vi "Save.vi"(8 "error in (no error)":errorcluster, 10 "File Path":path, 11 "Excel in":refnum<class "Excel.lvclass">) -> (0 "error out":errorcluster, 2 "Cancelled?":bool, 3 "Excel out":refnum<class "Excel.lvclass">)   [LabVIEW 2016, in "Excel.lvclass"]
doc: "Saves the Excel workbook referenced by the Excel input class.\n\nIf a file path is provided the workbook will be saved to that path overwriting existing files.\nIf a file path is not provided but the workbook has previously been saved the workbook will be saved to it's existing location.\nIf neither of the above are true the user will be prompted for a file path and if a file already exists at that path will be prompted again to ensure they want to overwrite the existing file.\n\nCancelled is returned as true if the file is not saved for any reason including an input error."
uses:
  Excel.lvclass
  Excel.lvclass/Excel.ctl
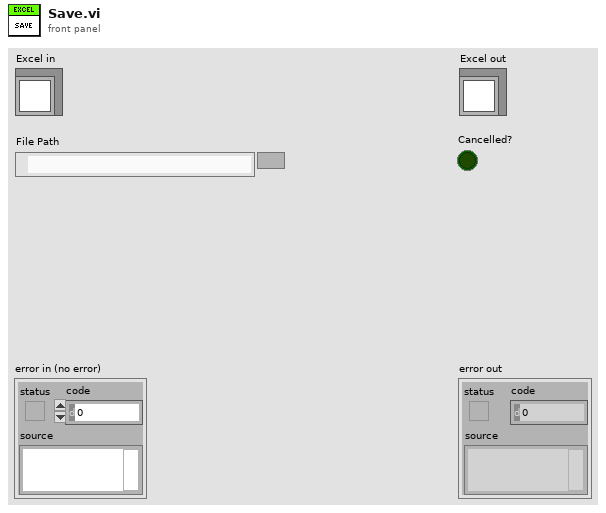
[diagram p1: front panel]
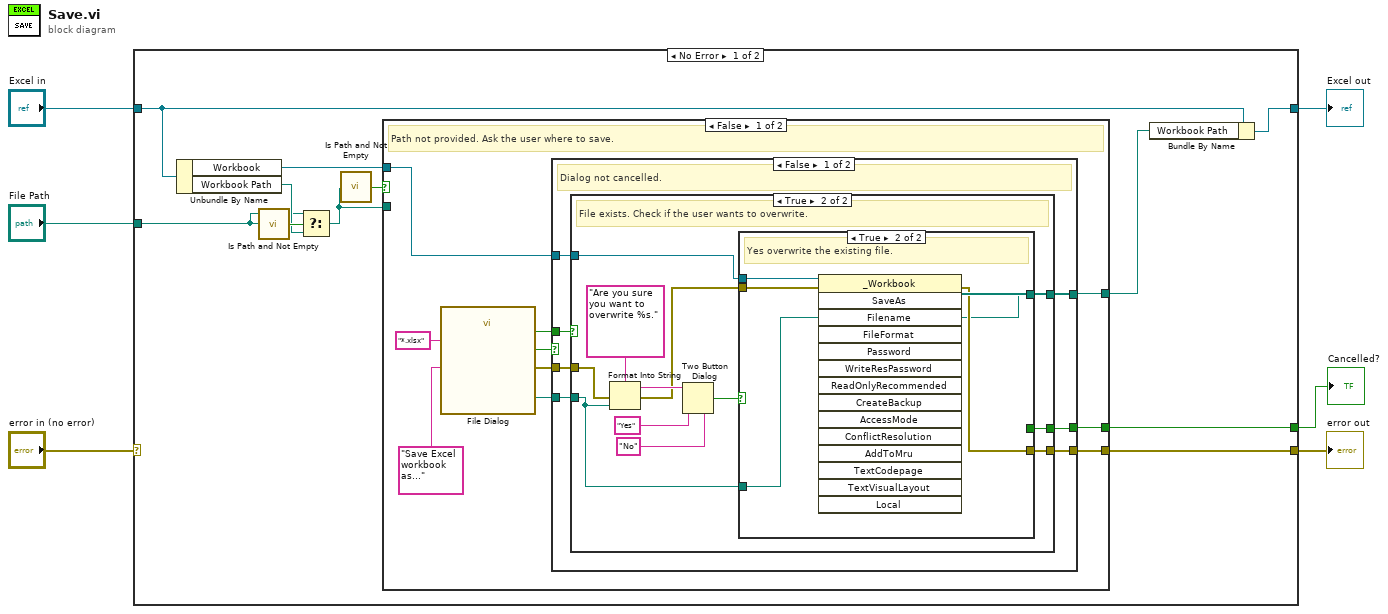
[diagram p0: block diagram]
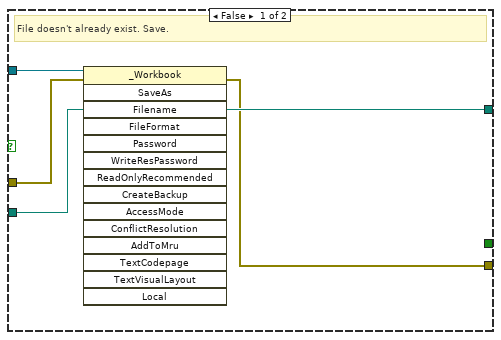
[diagram p2: hidden frame]
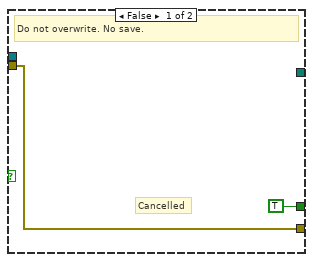
[diagram p3: hidden frame]
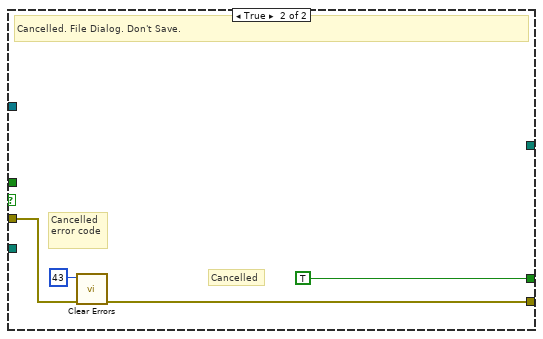
[diagram p4: hidden frame]
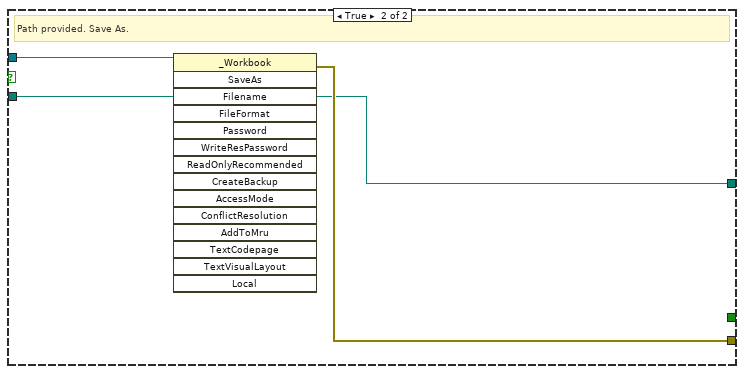
[diagram p5: hidden frame]
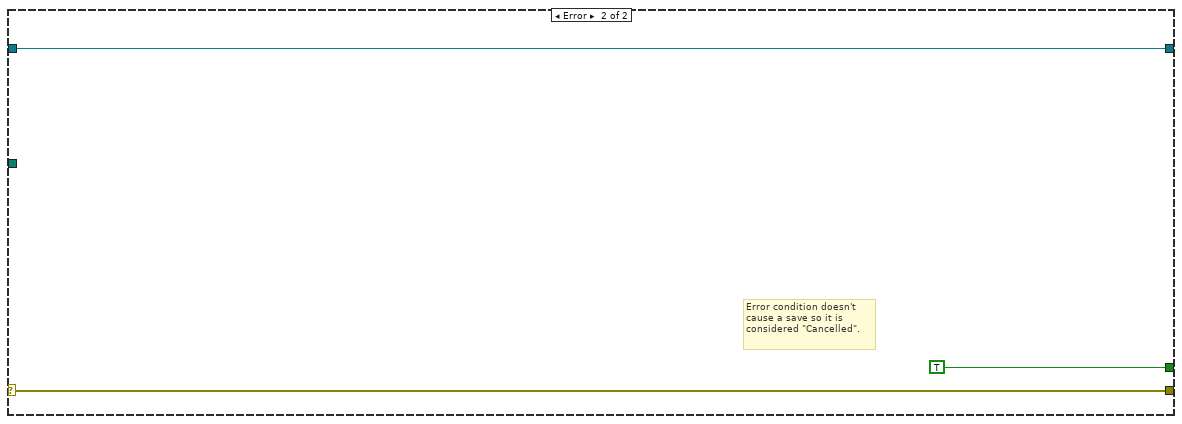
[diagram p6: hidden frame]
diagram:
  n1 = case shown="No Error" "error in (no error)" {
    selector: "error in (no error)" -> [_ w66]
    tunnel: [w13 w66] -> w5
    tunnel: [w16 w65] -> w3
    tunnel: "Excel in" -> [w17 w65]
    tunnel: "File Path" -> [w10 _]
    tunnel: [w7 TRUE] -> w1
    frame No Error {
      n2 = Unbundle By Name(w17) -> ("Workbook"=w15:refnum<k7>, "Workbook Path"=w11:path)
      n3 = call <vilib>:"Is Path and Not Empty.vi"("path"=w10) -> ("Is Path and Not Empty?"=w12:bool)  [unwired: 4 in]
      n4 = Select(t=w10, s=w12, f=w11) -> (s? t:f=w9:path)
      n5 = call <vilib>:"Is Path and Not Empty.vi"("path"=w9) -> ("Is Path and Not Empty?"=w8:bool)  [unwired: 4 in]
      n6 = case shown="False" w8 {
        tunnel: w15 -> [w18 w63]
        tunnel: w9 -> [_ w61]
        tunnel: [w22 w62] -> w13
        tunnel: [w21 w61] -> w14
        tunnel: [w20 _] -> w7
        frame False {
          # "Path not provided. Ask the user where to save."
          n7 = call "File Dialog"("prompt"="Save Excel workbook as..." ("pattern (all files)"), "pattern (all files)"="*.xlsx") -> ("selected path"=w19:path, "exists"=w24:bool, "cancelled"=w25:bool, "error out"=w23:errorcluster)  [unwired: 10 in]
          n8 = case shown="False" w25 {
            tunnel: w24 -> [w34 _]
            tunnel: w23 -> [w32 w60]
            tunnel: [w29 w58] -> w22
            tunnel: [w28 TRUE] -> w20
            tunnel: [w30 _] -> w21
            tunnel: w19 -> [w33 _]
            tunnel: w18 -> [w31 _]
            frame False {
              # "Dialog not cancelled."
              n9 = case shown="True" w34 {
                tunnel: w33 -> [w36 w40]
                tunnel: w32 -> [w38 w49]
                tunnel: w31 -> [w37 w44]
                tunnel: [w36 w39] -> w30
                tunnel: [w35 w42] -> w29
                tunnel: [_ w45] -> w28
                frame False {
                  # "File doesn't already exist. Save."
                  n10 = invoke class="_Workbook" method="SaveAs"(reference=w37, error in=w38, "Filename"=w36) -> (error out=w35:errorcluster)  [unwired: 12 in, 14 out]
                }
                frame True {
                  # "File exists. Check if the user wants to overwrite."
                  n11 = Format Into String(format string="Are you sure you want to overwrite %s." ("message"), error in=w49, w40) -> (resulting string=w46:string, error out=w43:errorcluster)  [unwired: 1 in]
                  n12 = Two Button Dialog(message=w46, 1:"No" ("T button name (\"OK\")"), 2:"Yes" ("T button name (\"OK\")")) -> (T button?=w41:bool)
                  n13 = case shown="True" w41 {
                    tunnel: [TRUE _] -> w45
                    tunnel: w44 -> [_ w56]
                    tunnel: w43 -> [w51 w55]
                    tunnel: [w51 w54] -> w42
                    tunnel: w40 -> [_ w53]
                    tunnel: [_ w53] -> w39
                    frame False {
                      # "Cancelled"
                      # "Do not overwrite. No save."
                    }
                    frame True {
                      # "Yes overwrite the existing file."
                      n14 = invoke class="_Workbook" method="SaveAs"(reference=w56, error in=w55, "Filename"=w53) -> (error out=w54:errorcluster)  [unwired: 12 in, 14 out]
                    }
                  }
                }
              }
            }
            frame True {
              # "Cancelled"
              # "Cancelled error code"
              # "Cancelled. File Dialog. Don't Save."
              n15 = call <vilib>:"Clear Errors.vi"("error in (no error)"=w60, "specific error code to clear (0: all)"=43) -> ("error out"=w58:errorcluster)  [unwired: 4 in, 1 out]
            }
          }
        }
        frame True {
          # "Path provided. Save As."
          n16 = invoke class="_Workbook" method="SaveAs"(reference=w63, "Filename"=w61) -> (error out=w62:errorcluster)  [unwired: 13 in, 14 out]
        }
      }
      n17 = Bundle By Name(cluster=w17, "Workbook Path"=w14) -> (w16:refnum<class "Excel.lvclass">)
    }
    frame Error {
      # "Error condition doesn't cause a save so it is considered \"Cancelled\"."
    }
  }
  "error out" <- w5
  "Excel out" <- w3
  "Cancelled?" <- w1
